vi "Msg.vi"(7 "Actor in":refnum<class "Actor.lvclass">, 11 "Destroy Msg in":refnum<class "Destroy Msg.lvclass">) -> (0 "Error out":errorcluster, 5 "Actor out":refnum<class "Actor.lvclass">)   [LabVIEW 2025, in "jettl.lvlib" / "Destroy Msg.lvlib" / "Destroy Msg.lvclass"]
uses:
  Destroy Msg.lvclass
  Destroy Msg.lvclass/Destroy Msg.ctl
  Destroy/Destroy.lvclass
  Actor/Actor/Actor.lvclass
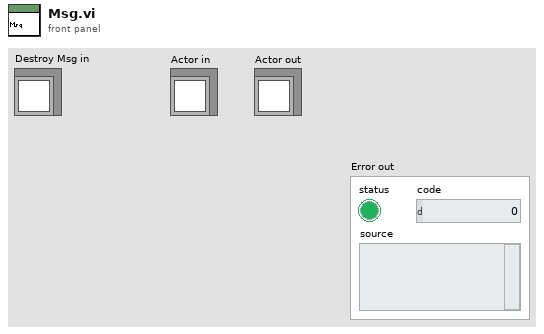
[diagram p1: front panel]
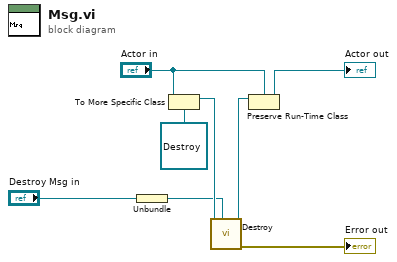
[diagram p0: block diagram]
diagram:
  n1 = Unbundle "Unbundle"("Destroy Msg in") -> (w2:refnum<class "Sender.lvclass">)
  n2 = To More Specific Class(target class=refnum<class "Destroy.lvclass"> refnum ("Destroy.lvlib:Destroy.lvclass"), reference="Actor in") -> (specific class reference=w4:refnum<class "Destroy.lvclass">)  [unwired: 1 in, 1 out]
  n3 = call-dynamic "Destroy.vi"("Sender"=w2, "Destroy in"=w4) -> ("Error out"=→"Error out":errorcluster, "Destroy out"=w3:refnum<class "Destroy.lvclass">)  [unwired: 8 in]
  n4 = Preserve Run-Time Class(object in=w3, 2:"Actor in") -> (object out=→"Actor out":refnum<class "Actor.lvclass">)  [unwired: 1 in, 1 out]
